vi "GetUnit.vi"(8 "error in (no error)":errorcluster, 11 "VISA resource name":refnum<visa-resource-name>="COM3") -> (0 "error out":errorcluster, 2 "Unit":u16(ring) items=["cm", "inch", "%"])   [LabVIEW 2017]
uses:
  <vilib>/Instr/_visa.llb/VISA Configure Serial Port (Instr).vi
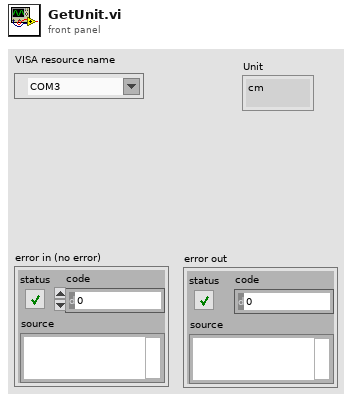
[diagram p1: front panel]
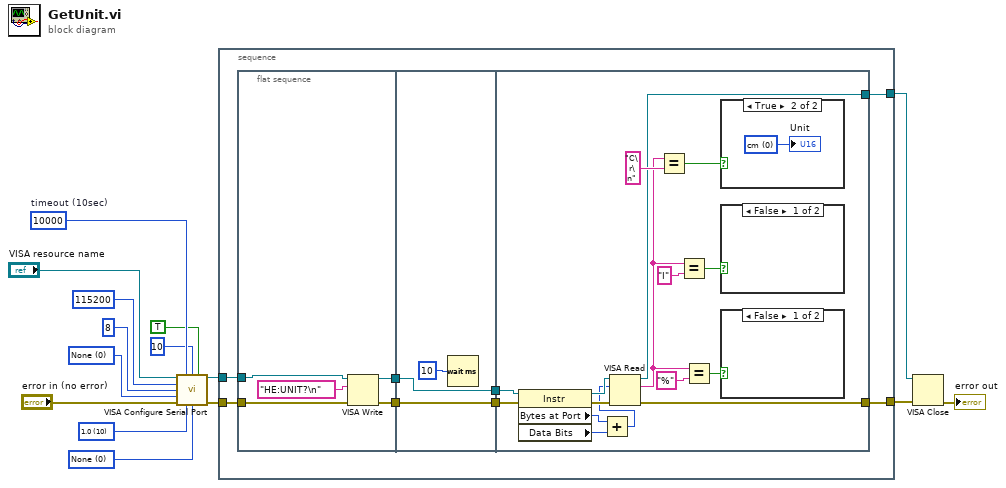
[diagram p0: block diagram]
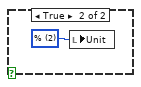
[diagram p2: hidden frame]
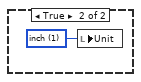
[diagram p3: hidden frame]
diagram:
  w5 = u16 0 items=["None"=0, "XON/XOFF"=1, "RTS/CTS"=2, "DTR/DSR"=4] ("flow control")
  w6 = u16 10 items=["1.0"=10, "1.5"=15, "2.0"=20] ("stop bits")
  w8 = u16 0 items=["None", "Odd", "Even", "Mark", "Space"] ("parity")
  w13 = u32 10000  # timeout (10sec)
  n1 = call-poly "VISA Configure Serial Port"("VISA resource name"="VISA resource name", "timeout (10sec)"=w13, "termination char\n(0xA = '\\n' = LF)"=u8 10 ("termination char\n(0xA = '\\n' = LF)"), "Enable Termination\nChar (T)"=TRUE ("Enable Termination Char (T)"), "baud rate (9600)"=u32 115200 ("baud rate"), "data bits (8)"=u16 8 ("data bits"), "parity (0:none)"=w8, "error in (no error)"="error in (no error)", "stop bits (10: 1 bit)"=w6, "flow control (0:none)"=w5) -> ("VISA resource name out"=w4:refnum<visa-resource-name>, "error out"=w3:errorcluster)  [unwired: 4 in]
  n2 = stacked-sequence {
    tunnel: w4 -> [w19]
    tunnel: w3 -> [w18]
    tunnel: [w17] -> w1
    tunnel: [w16] -> w2
    frame #0 {
      n3 = flat-sequence {
        tunnel: [w28] -> w23
        tunnel: [w27] -> w22
        tunnel: w19 -> [w25]
        tunnel: w18 -> [w24]
        tunnel: w23 -> [w31]
        tunnel: [w31] -> w21
        tunnel: w22 -> [w30]
        tunnel: [w30] -> w20
        tunnel: w21 -> [w47]
        tunnel: w20 -> [w46]
        tunnel: [w36] -> w16
        tunnel: [w35] -> w17
        frame #0 {
          n4 = VISA Write(VISA resource name=w25, write buffer="HE:UNIT?\n" ("string to write 2"), error in (no error)=w24) -> (VISA resource name out=w28:refnum<visa-resource-name>, error out=w27:errorcluster)  [unwired: 1 out]
        }
        frame #1 {
          n5 = Wait (ms)(milliseconds to wait=u32 10) -> ()  [unwired: 1 out]
        }
        frame #2 {
          n6 = property class="Instr"(reference=w47, error in=w46) -> (reference out=w44:refnum<visa-resource-name>, error out=w45:errorcluster, "Bytes at Port"=w34:u32, "Data Bits"=w33:u16)
          n7 = Add(x=w34, y=w33) -> (x+y=w32:u32)
          n8 = VISA Read(VISA resource name=w44, byte count=w32, error in (no error)=w45) -> (VISA resource name out=w35:refnum<visa-resource-name>, read buffer=w39:string, error out=w36:errorcluster)  [unwired: 1 out]
          n9 = Equal?(x=w39, y="C\r\n" ("read string")) -> (x = y?=w42:bool)
          n10 = Equal?(x=w39, y="I" ("read string")) -> (x = y?=w40:bool)
          n11 = Equal?(x=w39, y="%" ("read string")) -> (x = y?=w37:bool)
          n12 = case shown="True" w42 {
            frame False {
            }
            frame True {
              w50 = u16 0 items=["cm", "inch", "%"] ("Unit 2")
              "Unit" <- w50
            }
          }
          n13 = case shown="False" w40 {
            frame False {
            }
            frame True {
              w49 = u16 1 items=["cm", "inch", "%"] ("Unit 2")
              n14 = local write "Unit"(w49) -> ()
            }
          }
          n15 = case shown="False" w37 {
            frame False {
            }
            frame True {
              w48 = u16 2 items=["cm", "inch", "%"] ("Unit 2")
              n16 = local write "Unit"(w48) -> ()
            }
          }
        }
      }
    }
  }
  n17 = VISA Close(VISA resource name=w1, error in (no error)=w2) -> (error out=→"error out":errorcluster)
